vi "Cleanup Session.vi"(8 "error in (no error)":errorcluster, 11 "RandomNumberLogger in":refnum<class "RandomNumberLogger.lvclass">) -> (0 "error out":errorcluster, 3 "RandomNumberLogger out":refnum<class "RandomNumberLogger.lvclass">)   [LabVIEW 2020, in "RandomNumberLogger.lvlib" / "RandomNumberLogger.lvclass"]
doc: "<b>Cleanup Session</b>\nThis method is used to close any references opened in Configure Session and flush any buffers used.\n\nThis method is followed by either Configure Session (if the plugin is restarting) or Finalize (if the plugin is shutting down)."
uses:
  RandomNumberLogger.lvclass
  RandomNumberLogger.lvclass/RandomNumberLogger.ctl
  <vilib>/ADAS Record/Utilities/ADAS Utilities.lvlib
  C:/Program Files/National Instruments/LabVIEW 2020/vi.lib/FlexLogger/SDK/PluginSDK.lvlibp/PEFClasses/SDK/Processing Element/Processing Element.lvclass
  C:/Projects/GitHub/data-record-ad/IO Plugins/Tutorial Solutions/RandomNumberLogger/PE/RandomNumberLogger.lvclass
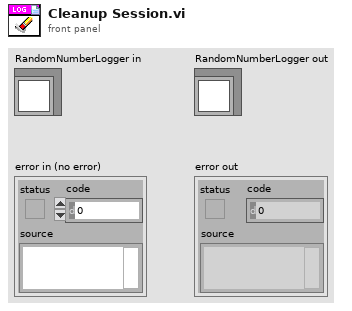
[diagram p1: front panel]
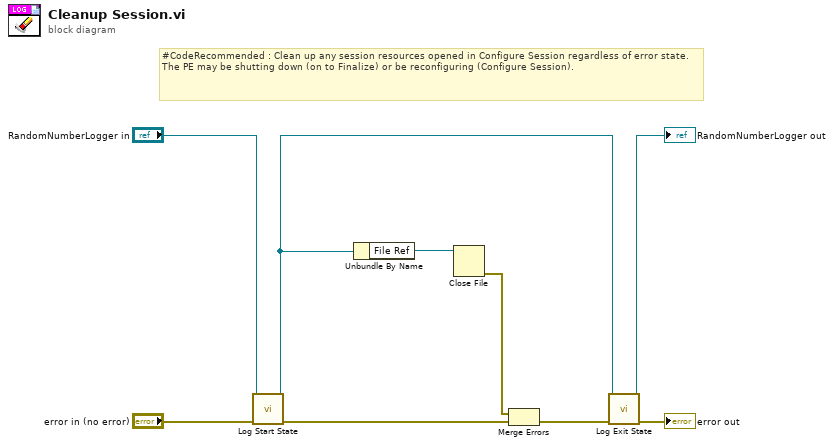
[diagram p0: block diagram]
diagram:
  # "#CodeRecommended : Clean up any session resources opened in Configure Session regardless of error state. The PE may be shutting down (on to Finalize) or be reconfiguring (Configure Session)."
  n1 = call <vilib>:"Log Start State.vi"("error in (no error)"="error in (no error)", "PluginSDK.lvlibp:Processing Element.lvclass"="RandomNumberLogger in") -> ("error out"=w8:errorcluster, "PluginSDK.lvlibp:Processing Element.lvclass"=w3:refnum<class "RandomNumberLogger.lvclass">)  [unwired: 8 in]
  n2 = Unbundle By Name(w3) -> ("File Ref"=w1:refnum<file>)
  n3 = Close File(refnum=w1) -> (error out=w2:errorcluster)  [unwired: 1 in, 1 out]
  n4 = Merge Errors(w2, w8) -> (w6:errorcluster)
  n5 = call <vilib>:"Log Exit State.vi"("error in (no error)"=w6, "PluginSDK.lvlibp:Processing Element.lvclass"=w3) -> ("error out"=→"error out":errorcluster, "PluginSDK.lvlibp:Processing Element.lvclass"=→"RandomNumberLogger out":refnum<class "RandomNumberLogger.lvclass">)  [unwired: 8 in]
